vi "Process Tab Key.vi"(0 "Back":refnum<vi>, 1 "Shift":bool, 2 "Char":i16, 5 "Next":refnum<vi>, 9 "Help":refnum<vi>, 12 "CurPage Ctrl #1":refnum<vi>, 13 "CurPage Ctrl #n":refnum<vi>) -> (4 "Discard Key Down Event?":bool)   [LabVIEW 2016]
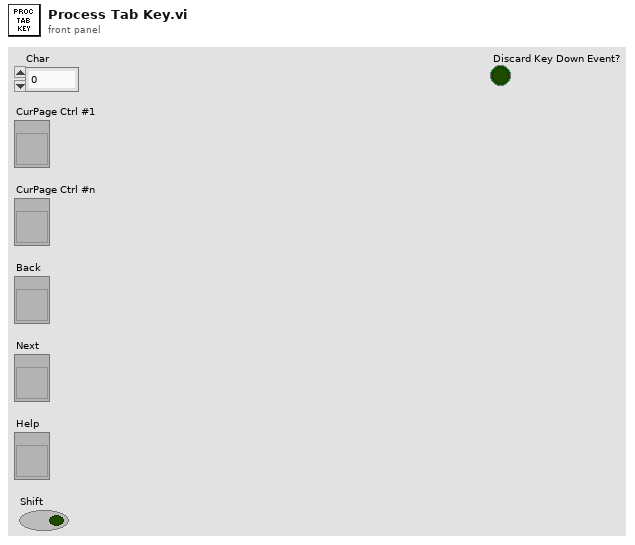
[diagram p1: front panel]
types:
  T1 = enum8{"Enabled", "Disabled", "Disabled and Grayed Out"}
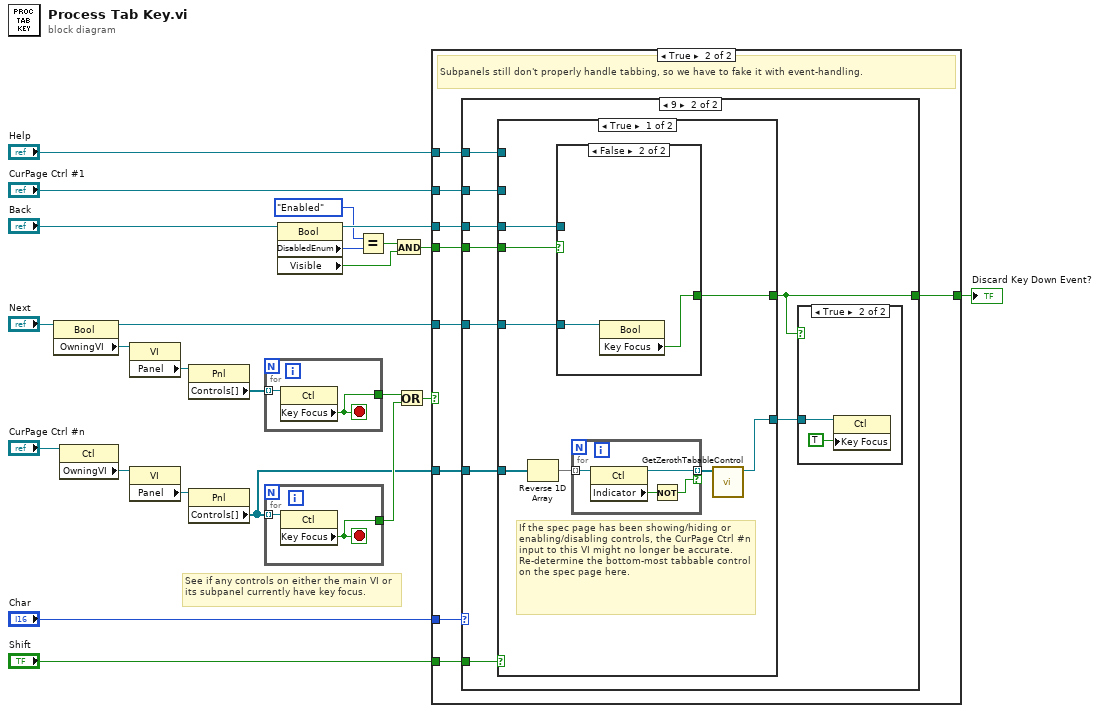
[diagram p0: block diagram]
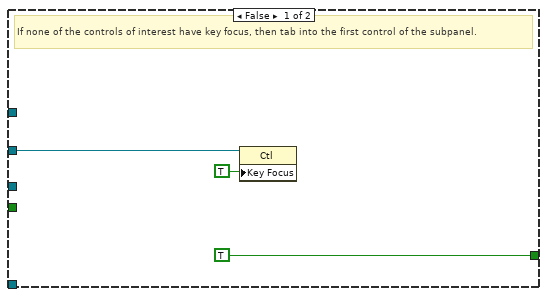
[diagram p2: hidden frame]
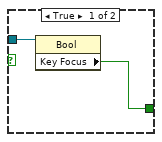
[diagram p5: hidden frame]
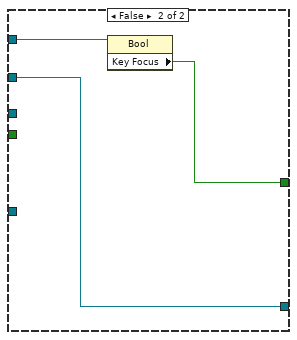
[diagram p6: hidden frame]
diagram:
  # "See if any controls on either the main VI or its subpanel currently have key focus."
  n1 = property class="Bool"(reference="Next") -> (reference out=w10:refnum<vi>, "OwningVI"=w9:refnum<vi>)  [unwired: 1 in, 1 out]
  n2 = property class="Ctl"(reference="CurPage Ctrl #n") -> ("OwningVI"=w5:refnum<vi>)  [unwired: 1 in, 2 out]
  n3 = property class="VI"(reference=w9) -> ("Panel"=w8:refnum<vi>)  [unwired: 1 in, 2 out]
  n4 = property class="VI"(reference=w5) -> ("Panel"=w6:refnum<vi>)  [unwired: 1 in, 2 out]
  n5 = property class="Pnl"(reference=w8) -> ("Controls[]"=w7:refnum<vi>[])  [unwired: 1 in, 2 out]
  n6 = property class="Pnl"(reference=w6) -> ("Controls[]"=w1:refnum<vi>[])  [unwired: 1 in, 2 out]
  n7 = for {
    tunnel: w7 -> [w26] mode=indexing
    tunnel: [w25] -> w3
    stop <- w25 stop-if-true
    n8 = property class="Ctl"(reference=w26) -> ("Key Focus"=w25:bool)  [unwired: 1 in, 2 out]
  }
  n9 = for {
    tunnel: w1 -> [w28] mode=indexing
    tunnel: [w27] -> w4
    stop <- w27 stop-if-true
    n10 = property class="Ctl"(reference=w28) -> ("Key Focus"=w27:bool)  [unwired: 1 in, 2 out]
  }
  n11 = property on="Property Node" class="Bool"(reference="Back") -> (reference out=w20:refnum<vi>, "DisabledEnum"=w14:T1, "Visible"=w17:bool)  [unwired: 1 in, 1 out]
  n12 = Equal?(x=T1."Enabled", y=w14) -> (x = y?=w16:bool)
  n13 = And(x=w16, y=w17) -> (x .and. y?=w18:bool)
  n14 = Or(x=w3, y=w4) -> (x .or. y?=w2:bool)
  n15 = case shown="True" w2 {
    tunnel: "CurPage Ctrl #1" -> [w31 w40]
    tunnel: "Help" -> [_ w39]
    tunnel: w10 -> [_ w38]
    tunnel: w20 -> [_ w37]
    tunnel: w18 -> [_ w36]
    tunnel: [TRUE ("Key Focus") w35] -> w13
    tunnel: "Shift" -> [_ w34]
    tunnel: "Char" -> [_ w33]
    tunnel: w1 -> [_ w32]
    frame False {
      # "If none of the controls of interest have key focus, then tab into the first control of the subpanel."
      n16 = property class="Ctl"(reference=w31, "Key Focus"=TRUE) -> ()  [unwired: 1 in, 2 out]
    }
    frame True {
      # "Subpanels still don't properly handle tabbing, so we have to fake it with event-handling."
      n17 = case shown="9" w33 {
        tunnel: w34 -> [_ w49]
        tunnel: [_ w48] -> w35
        tunnel: w36 -> [_ w46]
        tunnel: w37 -> [_ w45]
        tunnel: w38 -> [_ w44]
        tunnel: w39 -> [_ w43]
        tunnel: w40 -> [_ w42]
        tunnel: w32 -> [_ w41]
        frame Default {
        }
        frame 9 {
          n18 = case shown="True" w49 {
            tunnel: [w58 w70] -> w48
            tunnel: [w52 w68] -> w47
            tunnel: w46 -> [w59 _]
            tunnel: w45 -> [w57 _]
            tunnel: w44 -> [w56 _]
            tunnel: w43 -> [_ w69]
            tunnel: w42 -> [_ w68]
            tunnel: w41 -> [w55 _]
            frame True {
              # "If the spec page has been showing/hiding or enabling/disabling controls, the CurPage Ctrl #n input to this VI might no longer be accurate. Re-determine the bottom-most tabbable control on the spec page here."
              n19 = Reverse 1D Array(array=w55) -> (reversed array=w54:refnum<vi>[])
              n20 = case shown="False" w59 {
                tunnel: [w65 w67] -> w58
                tunnel: w57 -> [w64 _]
                tunnel: w56 -> [_ w66]
                frame True {
                  n21 = property on="Property Node" class="Bool"(reference=w64) -> ("Key Focus"=w65:bool)  [unwired: 1 in, 2 out]
                }
                frame False {
                  n22 = property on="Property Node" class="Bool"(reference=w66) -> ("Key Focus"=w67:bool)  [unwired: 1 in, 2 out]
                }
              }
              n23 = for {
                tunnel: w54 -> [w63] mode=indexing
                tunnel: [w62] -> w53 mode=indexing if=w60
                n24 = property class="Ctl"(reference=w63) -> (reference out=w62:refnum<vi>, "Indicator"=w61:bool)  [unwired: 1 in, 1 out]
                n25 = Not(x=w61) -> (.not. x?=w60:bool)
              }
              n26 = call <resource>:"GetZerothTabableControl.vi"("Controls[]"=w53) -> ("Control out"=w52:refnum<vi>)  [unwired: 10 in]
            }
            frame False {
              n27 = property on="Property Node" class="Bool"(reference=w69) -> ("Key Focus"=w70:bool)  [unwired: 1 in, 2 out]
            }
          }
          n28 = case shown="True" w48 {
            tunnel: w47 -> [_ w50]
            frame False {
            }
            frame True {
              n29 = property on="Property Node" class="Ctl"(reference=w50, "Key Focus"=TRUE) -> ()  [unwired: 1 in, 2 out]
            }
          }
        }
      }
    }
  }
  "Discard Key Down Event?" <- w13
